vi "Subvi pixel clock gated.vi"(5 "Nmax lines":u16, 7 "Start_acquisition":bool, 11 "Pixel clock/line clock change":T1) -> (0 "Line clock start":bool, 1 "Gated pixel clock change":bool)   [LabVIEW 2017]
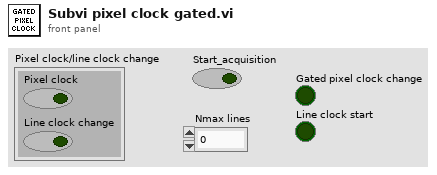
[diagram p1: front panel]
types:
  T1 = cluster{"Pixel clock":bool, "Line clock change":bool}
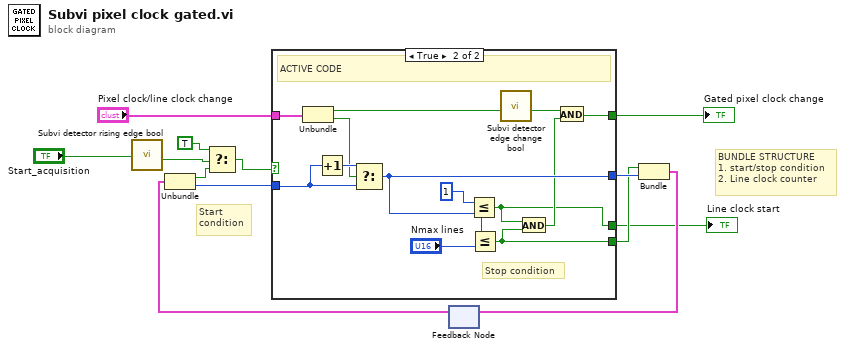
[diagram p0: block diagram]
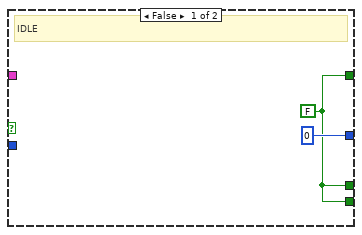
[diagram p2: hidden frame]
diagram:
  # "Start\ncondition"
  # "BUNDLE STRUCTURE\n1. start/stop condition\n2. Line clock counter"
  n1 = call "Subvi detector rising edge bool.vi"("Input"="Start_acquisition") -> ("Output"=w3:bool)  [unwired: 10 in]
  n2 = feedback #1() -> (w11:cluster{bool, u16})  [unwired: 1 in]
  n3 = Unbundle(w11) -> (w12:bool, w13:u16)
  n4 = Select(t=TRUE, s=w3, f=w12) -> (s? t:f=w7:bool)
  n5 = case shown="True" w7 {
    tunnel: [w14 w19] -> w8
    tunnel: w13 -> [_ w28]
    tunnel: [u16 0 w27] -> w9
    tunnel: "Pixel clock/line clock change" -> [_ w26]
    tunnel: [w14 w24] -> w2
    tunnel: [w14 w16] -> w1
    frame False {
      w14 = FALSE
      # "IDLE"
    }
    frame True {
      # "Stop condition"
      # "ACTIVE CODE"
      n6 = Unbundle(w26) -> ("Pixel clock"=w20:bool, "Line clock change"=w17:bool)
      n7 = Increment(x=w28) -> (x+1=w23:u16)
      n8 = Select(t=w23, s=w17, f=w28) -> (s? t:f=w27:u16)
      n9 = Less Or Equal?(x=u16 1 ("Min"), y=w27) -> (x <= y?=w16:bool)
      n10 = Less Or Equal?(x=w27, y="Nmax lines") -> (x <= y?=w19:bool)
      n11 = call "Subvi detector edge change bool.vi"("Input"=w20) -> ("Output"=w21:bool)  [unwired: 8 in]
      n12 = And(x=w16, y=w19) -> (x .and. y?=w18:bool)
      n13 = And(x=w21, y=w18) -> (x .and. y?=w24:bool)
    }
  }
  "Gated pixel clock change" <- w2
  "Line clock start" <- w1
  n14 = Bundle(w8, w9) -> (w10:cluster{bool, u16})  [unwired: 1 in]
  n15 = feedback-in #1(w10) -> ()
